vi "Double Structure.vi"(1 "change":string, 2 "-+ structure":string, 3 "string":string) -> (0 "- structure":string)   [LabVIEW 2020, in "NI_Gmath.lvlib"]
uses:
  <vilib>/gmath/NI_Gmath.lvlib
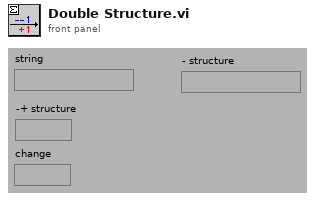
[diagram p1: front panel]
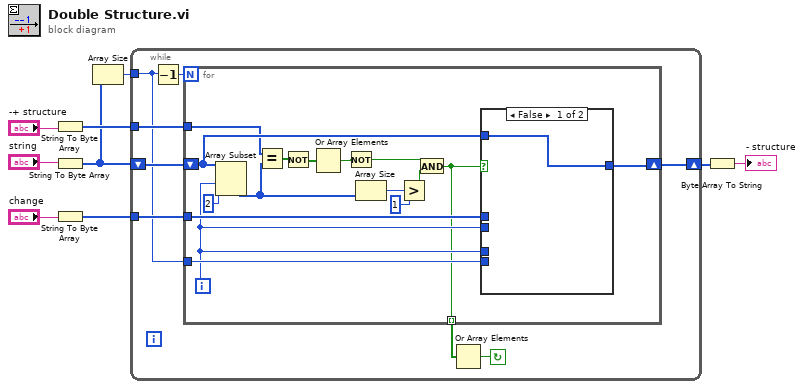
[diagram p0: block diagram]
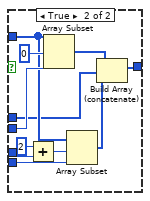
[diagram p2: hidden frame]
diagram:
  n1 = String To Byte Array(string="-+ structure") -> (unsigned byte array=w9:u8[])
  n2 = String To Byte Array(string="string") -> (unsigned byte array=w1:u8[])
  n3 = String To Byte Array(string="change") -> (unsigned byte array=w7:u8[])
  n4 = Array Size(array=w1) -> (size(s)=w6:i32)
  n5 = while {
    tunnel: w6 -> [w14]
    tunnel: w7 -> [w15]
    tunnel: w9 -> [w16]
    shift-left: w1 -> [w17]
    shift-right: [w10] -> w2
    stop <- w12 continue-if-true
    n6 = Decrement(x=w14) -> (x-1=w11:i32)
    n7 = for {
      N: w11 -> [_]
      shift-right: [w25] -> w10
      shift-left: w17 -> [w32]
      tunnel: w16 -> [w23]
      tunnel: w15 -> [w31]
      tunnel: w14 -> [w30]
      tunnel: [w24] -> w13 mode=indexing
      i -> [w29]
      n8 = Array Subset(array=w32, index=w29, length=2) -> (w22:u8[])
      n9 = Equal?(x=w23, y=w22) -> (x = y?=w21:bool[])
      n10 = Not(x=w21) -> (.not. x?=w18:bool[])
      n11 = Or Array Elements(Boolean array=w18) -> (logical OR=w20:bool)
      n12 = Not(x=w20) -> (.not. x?=w19:bool)
      n13 = Array Size(array=w22) -> (size(s)=w28:i32)
      n14 = Greater?(x=w28, y=1) -> (0:w26:bool)
      n15 = And(x=w19, y=w26) -> (x .and. y?=w24:bool)
      n16 = case shown="False" w24 {
        tunnel: w32 -> [w34 w41]
        tunnel: [w34 w45] -> w25
        tunnel: w29 -> [_ w42]
        tunnel: w31 -> [_ w35]
        tunnel: w30 -> [_ w40]
        tunnel: w29 -> [_ w39]
        frame False {
        }
        frame True {
          n17 = Add(x=2, y=w39) -> (x+y=w38:i32)
          n18 = Array Subset(array=w41, index=0, length=w42) -> (w44:u8[])
          n19 = Array Subset(array=w41, index=w38, length=w40) -> (w36:u8[])
          n20 = Build Array (concatenate)(w44, w35, w36) -> (w45:u8[])
        }
      }
    }
    n21 = Or Array Elements(Boolean array=w13) -> (logical OR=w12:bool)
  }
  n22 = Byte Array To String(unsigned byte array=w2) -> (string=→"- structure":string)
